vi "设置曲线属性.vi"(7 "XY图输入":refnum<vi>, 8 "错误输入（无错误）":errorcluster, 11 "曲线属性":T1[](array[typedef])=[{"曲线名"="上升过程", "曲线颜色"=0, "线条宽度"=2}, {"曲线名"="下降过程", "曲线颜色"=16711680, "线条宽度"=2}, {"曲线名"="3", "曲线颜色"=6618880, "线条宽度"=2}]) -> (0 "错误输出":errorcluster)   [LabVIEW 2020]
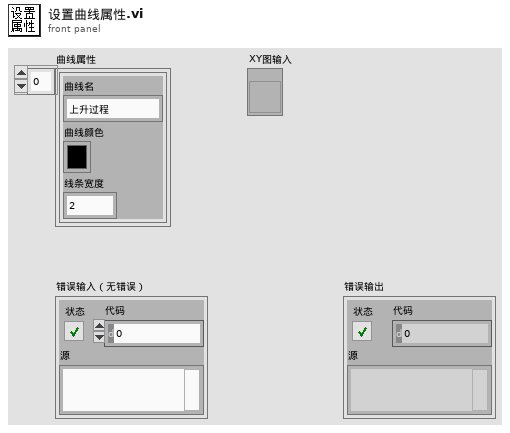
[diagram p1: front panel]
types:
  T1 = typedef "曲线属性.ctl" = cluster{"曲线名":string, "曲线颜色":u32, "线条宽度":u8}
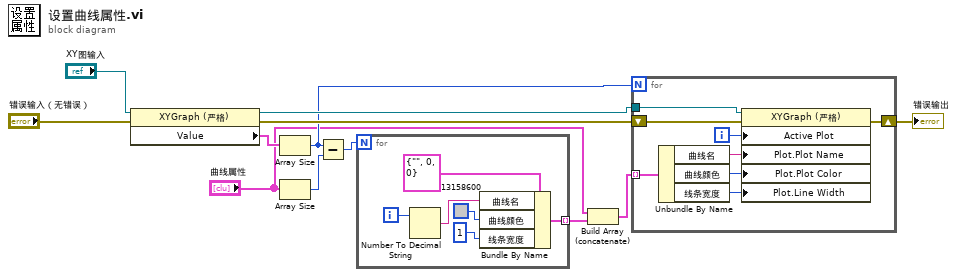
[diagram p0: block diagram]
diagram:
  n1 = property on="属性节点" class="XYGraph (严格)"(reference="XY图输入", error in="错误输入（无错误）") -> (reference out=w5:refnum<vi>, error out=w11:errorcluster, "Value"=w10:cluster{"测试数据":dbl[], "测试数据":dbl[]}[])
  n2 = Array Size(array=w10) -> (size(s)=w4:i32)
  n3 = Array Size(array="曲线属性") -> (size(s)=w3:i32)
  n4 = Subtract(x=w4, y=w3) -> (x-y=w2:i32)
  n5 = for {
    N: w2 -> [_]
    tunnel: [w14] -> w8 mode=indexing
    i -> [w15]
    n6 = Number To Decimal String(number=w15) -> (decimal integer string=w16:string)  [unwired: 1 in]
    n7 = Bundle By Name(cluster=T1 {"曲线名"="", "曲线颜色"=0, "线条宽度"=0} ("曲线属性"), "曲线名"=w16, "曲线颜色"=u32 13158600, "线条宽度"=u8 1) -> (w14:T1)
  }
  n8 = Build Array (concatenate)("曲线属性", w8) -> (w9:T1[])
  n9 = for {
    N: w4 -> [_]
    tunnel: w9 -> [w24] mode=indexing
    shift-right: [w21] -> w12
    shift-left: w11 -> [w22]
    tunnel: w5 -> [w20]
    i -> [w26]
    n10 = Unbundle By Name(w24) -> ("曲线名"=w25:string, "曲线颜色"=w23:u32, "线条宽度"=w19:u8)
    n11 = property on="属性节点" class="XYGraph (严格)"(reference=w20, error in=w22, "Active Plot"=w26, "Plot.Plot Name"=w25, "Plot.Plot Color"=w23, "Plot.Line Width"=w19) -> (error out=w21:errorcluster)  [unwired: 1 out]
  }
  "错误输出" <- w12
